vi "Configure Range Table (Spurious Emissions - Sweep And Limit).vi"(0 "VISA resource name":refnum<visa-resource-name>, 1 "Enable Auto Absolute Limit":bool[](array[boolean])=[TRUE, TRUE], 2 "Manual Absolute Stop Limit":dbl[](array[numeric])=[-50.0, -50.0] format="%#.6g", 5 "Sweep Time":dbl[](array[numeric])=[1.0, 1.0], 7 "Absolute Start Limit":dbl[](array[numeric])=[-49.0, -49.0] format="%#.6g", 11 "error in (no error)":errorcluster) -> (4 "VISA resource name out":refnum<visa-resource-name>, 15 "error out":errorcluster)   [LabVIEW 2014, in "Agilent ESA PSA Series.lvlib"]
doc: "Configures the sweeping paremeters of the measurement."
uses:
  Agilent ESA PSA Series.lvlib
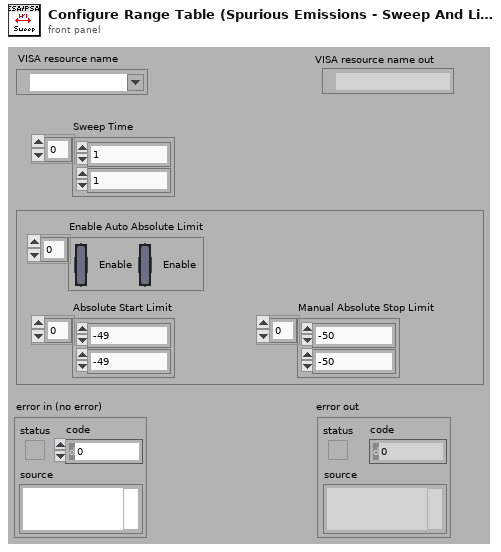
[diagram p1: front panel]
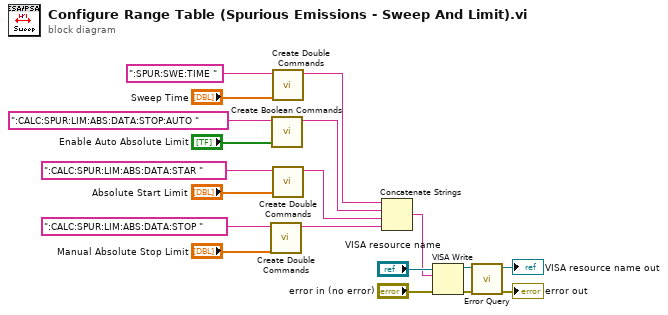
[diagram p0: block diagram]
diagram:
  n1 = call "Create Double Commands.vi"("Double Values"="Manual Absolute Stop Limit", "Commands"=":CALC:SPUR:LIM:ABS:DATA:STOP ") -> ("Result"=w5:string)  [unwired: 9 in]
  n2 = call "Create Boolean Commands.vi"("States"="Enable Auto Absolute Limit", "Command"=":CALC:SPUR:LIM:ABS:DATA:STOP:AUTO ") -> ("Result String"=w7:string)  [unwired: 9 in]
  n3 = call "Create Double Commands.vi"("Double Values"="Sweep Time", "Commands"=":SPUR:SWE:TIME ") -> ("Result"=w3:string)  [unwired: 9 in]
  n4 = call "Create Double Commands.vi"("Double Values"="Absolute Start Limit", "Commands"=":CALC:SPUR:LIM:ABS:DATA:STAR ") -> ("Result"=w6:string)  [unwired: 9 in]
  n5 = Concatenate Strings(w3, w7, w6, w5) -> (w4:string)
  n6 = VISA Write(VISA resource name="VISA resource name", write buffer=w4, error in (no error)="error in (no error)") -> (VISA resource name out=w2:refnum<visa-resource-name>, error out=w1:errorcluster)  [unwired: 1 out]
  n7 = call "Error Query.vi"("error in (no error)"=w1, "VISA resource name"=w2) -> ("error out"=→"error out":errorcluster, "VISA resource name out"=→"VISA resource name out":refnum<visa-resource-name>)  [unwired: 6 in, 2 out]
